vi "Main.vi"() -> ()   [LabVIEW 2019, in "LibraryTest.lvlib"]
uses:
  LibraryTest.lvlib
  <vilib>/numeric/Random Number (Range) DBL.vi
panel:
  out "Waveform Chart":dbl(graph)
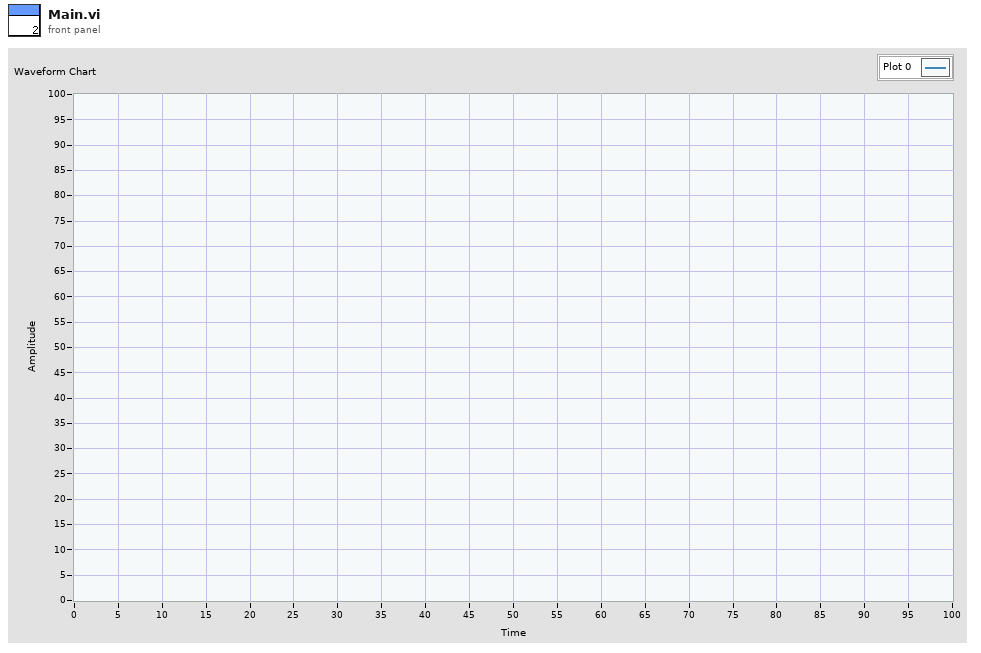
[diagram p1: front panel]
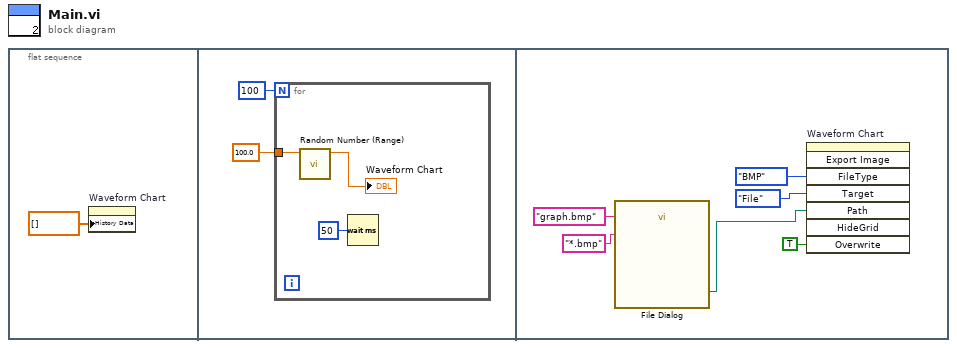
[diagram p0: block diagram]
diagram:
  n1 = flat-sequence {
    frame #0 {
      n2 = property on="Waveform Chart" class="WFChart (strict)"("History Data"=dbl[] []) -> ()  [unwired: 2 in, 2 out]
    }
    frame #1 {
      n3 = for {
        N: 100 -> [_]
        tunnel: 100.0 ("upper bound (100)") -> [w6]
        n4 = call-poly <vilib>:"Random Number (Range).vi"("upper bound (100)"=w6) -> ("number"=→"Waveform Chart":dbl)  [unwired: 10 in]
        n5 = Wait (ms)(milliseconds to wait=u32 50) -> ()  [unwired: 1 out]
      }
    }
    frame #2 {
      n6 = call "File Dialog"("default name"="graph.bmp", "pattern (all files)"="*.bmp" ("pattern label")) -> ("selected path"=w9:path)  [unwired: 10 in, 3 out]
      n7 = invoke on="Waveform Chart" class="WFChart (strict)" method="Export Image"("FileType"=enum32{"BMP", "EPS", "EMF", "PICT"}."BMP" ("File Type"), "Target"=enum32{"File", "Clipboard"}."File", "Path"=w9, "Overwrite"=TRUE ("Always Overwrite")) -> ()  [unwired: 4 in, 8 out]
    }
  }
